vi "Calc Traverse Components .vi"(11 "Traverse Robot":T1 {"Angle" scale format="%.3f"; "Velocity" scale=-1.0..1.0 scale format="%.1f"}) -> (3 "Swerve Data":T4 {"Back Right"."Angle" scale format="%.3f"; "Back Right"."Velocity" scale=-1.0..1.0 scale format="%.1f"; "Back Left"."Angle" scale format="%.3f"; "Back Left"."Velocity" scale=-1.0..1.0 scale format="%.1f"; "Front Left"."Angle" scale format="%.3f"; "Front Left"."Velocity" scale=-1.0..1.0 scale format="%.1f"; "Front Right"."Angle" scale format="%.3f"; "Front Right"."Velocity" scale=-1.0..1.0 scale format="%.1f"})   [LabVIEW 2020, in "SwerveDrive_ACT_ts.lvlib"]
uses:
  SwerveDrive_ACT_ts.lvlib
  Shared Code/TypeDefs/Cluster_Swerve 4 Steer and Velocity.ctl
  Shared Code/TypeDefs/Cluster_Module Velocity-Direction-Rotations.ctl
  Shared Code/TypeDefs/Level_Velocity plus-minus 1.ctl
  Shared Code/TypeDefs/Dial_Compase heading unit circle CCW positive.ctl
panel:
  # "\"Front\" of Robot"
  # "Right Hand Rule"
  # "X"
  # "+CCW"
  # "Y"
  # "(0,0)"
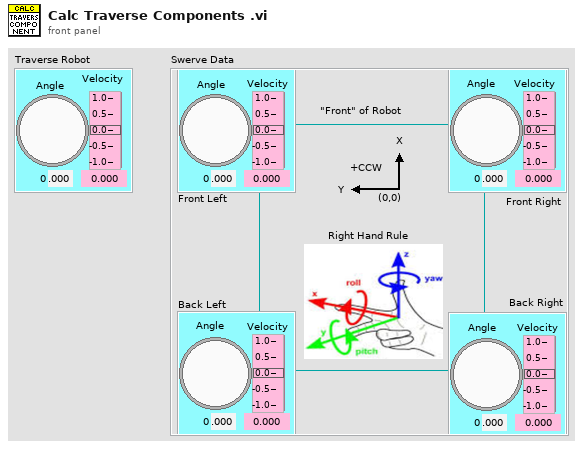
[diagram p1: front panel]
types:
  T1 = typedef "Cluster_Module Velocity-Direction-Rotations.ctl" = cluster{"Velocity":T2, "Angle":T3, "Rotations Count":dbl}
  T2 = typedef "Level_Velocity plus-minus 1.ctl" = dbl
  T3 = typedef "Dial_Compase heading unit circle CCW positive.ctl" = dbl
  T4 = typedef "Cluster_Swerve 4 Steer and Velocity.ctl" = cluster{"Front Right":T1, "Front Left":T1, "Back Left":T1, "Back Right":T1}
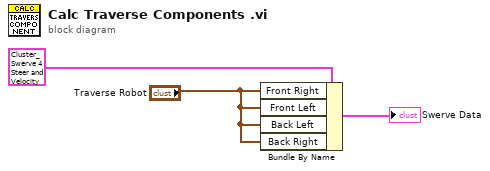
[diagram p0: block diagram]
diagram:
  n1 = Bundle By Name(cluster=T4 {"Front Right"={"Velocity"=0.0, "Angle"=0.0, "Rotations Count"=0.0}, "Front Left"={"Velocity"=0.0, "Angle"=0.0, "Rotations Count"=0.0}, "Back Left"={"Velocity"=0.0, "Angle"=0.0, "Rotations Count"=0.0}, "Back Right"={"Velocity"=0.0, "Angle"=0.0, "Rotations Count"=0.0}} ("Swerve Data"), "Front Right"="Traverse Robot", "Front Left"="Traverse Robot", "Back Left"="Traverse Robot", "Back Right"="Traverse Robot") -> (→"Swerve Data":T4)
